vi "RSZVB Get Calibration Auto Assignment Definition.vi"(0 "VISA resource name":refnum<visa-resource-name>, 5 "Channel (1)":i32=1, 7 "Assignment (1)":i32=1, 11 "error in (no error)":errorcluster {"code" format="%.0x"}) -> (2 "Cal Unit Port 3":i32, 3 "Cal Unit Port 1":i32, 4 "VISA resource name out":refnum<visa-resource-name>, 6 "Analyzer Port 1":i32, 8 "Analyzer Port 2":i32, 10 "Analyzer Port 3":i32, 12 "Cal Unit Port 4":i32, 13 "Cal Unit Port 2":i32, 14 "Analyzer Port 4":i32, 15 "error out":errorcluster {"code" format="%.0x"})   [LabVIEW 2011]
doc: "This VI queries a port assignment numbered <Assignment>. This command is particularly relevant for multiple port\nassignments.\n\nRemote-control command(s):\n[SENSe<Ch>:]CORRection:COLLect:AUTO:ASSignment<Asg>:DEFine?"
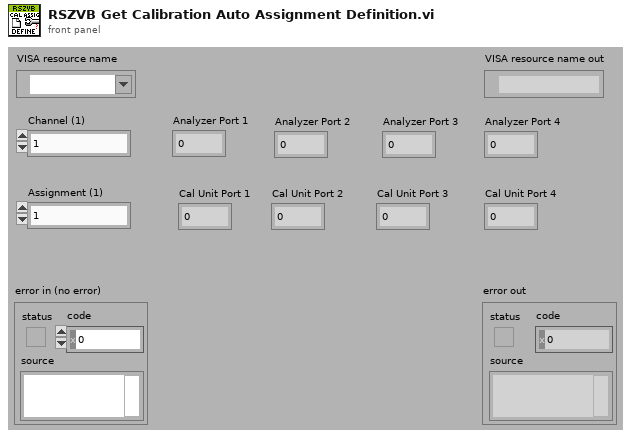
[diagram p1: front panel]
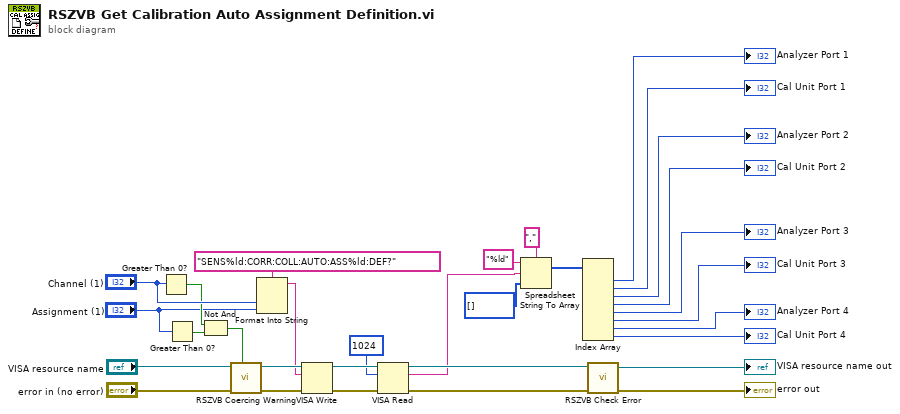
[diagram p0: block diagram]
diagram:
  n1 = Greater Than 0?(x="Channel (1)") -> (x > 0?=w19:bool)
  n2 = Greater Than 0?(x="Assignment (1)") -> (x > 0?=w17:bool)
  n3 = Not And(1:w17, 2:w19) -> (0:w16:bool)
  n4 = call "RSZVB Coercing Warning.vi"("In Range?"=w16, "error in (no error)"="error in (no error)", "VISA session"="VISA resource name") -> ("error out"=w30:errorcluster, "dup VISA session"=w31:refnum<visa-resource-name>)  [unwired: 7 in]
  n5 = Format Into String(format string="SENS%ld:CORR:COLL:AUTO:ASS%ld:DEF?", "Channel (1)", "Assignment (1)") -> (resulting string=w23:string)  [unwired: 2 in, 1 out]
  n6 = VISA Write(VISA resource name=w31, write buffer=w23, error in (no error)=w30) -> (VISA resource name out=w29:refnum<visa-resource-name>, error out=w28:errorcluster)  [unwired: 1 out]
  n7 = VISA Read(VISA resource name=w29, byte count=u32 1024 ("byte count (0)"), error in (no error)=w28) -> (VISA resource name out=w27:refnum<visa-resource-name>, read buffer=w1:string, error out=w26:errorcluster)  [unwired: 1 out]
  n8 = Spreadsheet String To Array(delimiter (Tab)=",", format string="%ld", spreadsheet string=w1, array type (2D Dbl)=i32[] []) -> (array=w12:i32[])
  n9 = Index Array(array=w12) -> (element #1=→"Analyzer Port 1":i32, element #2=→"Cal Unit Port 1":i32, element #3=→"Analyzer Port 2":i32, element #4=→"Cal Unit Port 2":i32, element #5=→"Analyzer Port 3":i32, element #6=→"Cal Unit Port 3":i32, element #7=→"Analyzer Port 4":i32, element #8=→"Cal Unit Port 4":i32)  [unwired: 8 in]
  n10 = call "RSZVB Check Error.vi"("error in (no error)"=w26, "VISA session"=w27) -> ("error out"=→"error out":errorcluster, "dup VISA session"=→"VISA resource name out":refnum<visa-resource-name>)  [unwired: 8 in]
